vi "Node Count.vi"(1 "Bus Number in":i32) -> (0 "Node Number":i32)   [LabVIEW 2014, in "Initialization and IO Node Scripting.lvlib"]
uses:
  Initialization and IO Node Scripting.lvlib
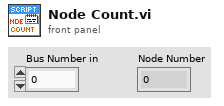
[diagram p1: front panel]
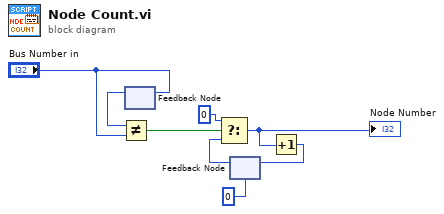
[diagram p0: block diagram]
diagram:
  n1 = feedback #1() -> (w2:i32)  [unwired: 1 in]
  n2 = Not Equal?(x=w2, y="Bus Number in") -> (x != y?=w4:bool)
  n3 = feedback-in #1("Bus Number in") -> ()
  n4 = feedback #2(0 ("Bus Number")) -> (w8:i32)
  n5 = Select(t=0 ("Bus Number"), s=w4, f=w8) -> (s? t:f=w6:i32)
  "Node Number" <- w6
  n6 = Increment(x=w6) -> (x+1=w7:i32)
  n7 = feedback-in #2(w7) -> ()
